vi "Helper - Parse Traverse Results.vi"(11 "Traverse Results":string[](array[string])) -> (3 "Parsed Results":string[][](array[string]))   [LabVIEW 2019]
doc: "This VI is used by the Using Traverse.vi example. Count the number of each unique class in the Traverse Results array, and generate a resulting array with those classes, and their number of occurrences."
panel:
  # "Count the number of each unique class in the Traverse Results array, and generate a resulting array with those classes, and their number of occurrences."
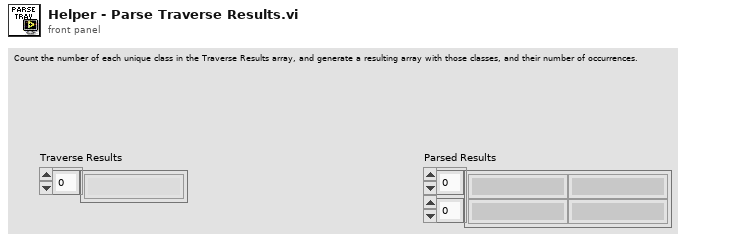
[diagram p1: front panel]
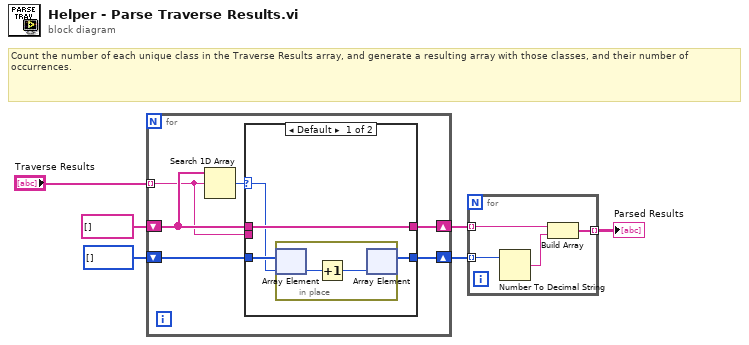
[diagram p0: block diagram]
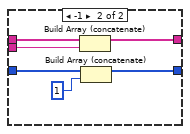
[diagram p2: hidden frame]
diagram:
  # "Count the number of each unique class in the Traverse Results array, and generate a resulting array with those classes, and their number of occurrences."
  n1 = for {
    tunnel: "Traverse Results" -> [w9] mode=indexing
    shift-right: [w10] -> w3
    shift-left: string[] [] -> [w11]
    shift-right: [w7] -> w2
    shift-left: i32[] [] -> [w8]
    n2 = Search 1D Array(1D array=w11, element=w9) -> (index of element=w12:i32)  [unwired: 1 in]
    n3 = case shown="Default" w12 {
      selector: w12 -> [w14 _]
      tunnel: w11 -> [w16 w24]
      tunnel: [w16 w22] -> w10
      tunnel: w9 -> [_ w23]
      tunnel: w8 -> [w15 w21]
      tunnel: [w13 w20] -> w7
      frame Default {
        n4 = in-place {
          n5 = in-place-array #1(w15, w14) -> (w18:i32)
          n6 = Increment(x=w18) -> (x+1=w17:i32)
          n7 = in-place-array #1(w17) -> (w13:i32[])  [unwired: 1 out]
        }
      }
      frame -1 {
        n8 = Build Array (concatenate)(w24, w23) -> (w22:string[])
        n9 = Build Array (concatenate)(w21, 1) -> (w20:i32[])
      }
    }
  }
  n10 = for {
    tunnel: w3 -> [w28] mode=indexing
    tunnel: w2 -> [w27] mode=indexing
    tunnel: [w25] -> w1 mode=indexing
    n11 = Number To Decimal String(number=w27) -> (decimal integer string=w26:string)  [unwired: 1 in]
    n12 = Build Array(w28, w26) -> (w25:string[])
  }
  "Parsed Results" <- w1
